vi "Sort queue by Time to next scan.vi"(4 "Queue":T1 {"Scan settings in queue" items=["Regular", "Inverted", "MartinaSettings"]; "Time of the last scan (s)" format="%<%H:%M:%S>t"; "When did you stick it in?" format="%<%H:%M:%S>t"; "Time to next scan (s)" format="%<%H:%M:%S>t"; "Time in rig (s)" format="%<%H:%M:%S>t"}) -> (1 "Queue Out":T1 {"Scan settings in queue" items=["Regular", "Inverted", "MartinaSettings"]; "Time of the last scan (s)" format="%<%H:%M:%S>t"; "When did you stick it in?" format="%<%H:%M:%S>t"; "Time to next scan (s)" format="%<%H:%M:%S>t"; "Time in rig (s)" format="%<%H:%M:%S>t"})   [LabVIEW 2011]
uses:
  Typedefs/Queue.ctl
  Typedefs/Queue cluster.ctl
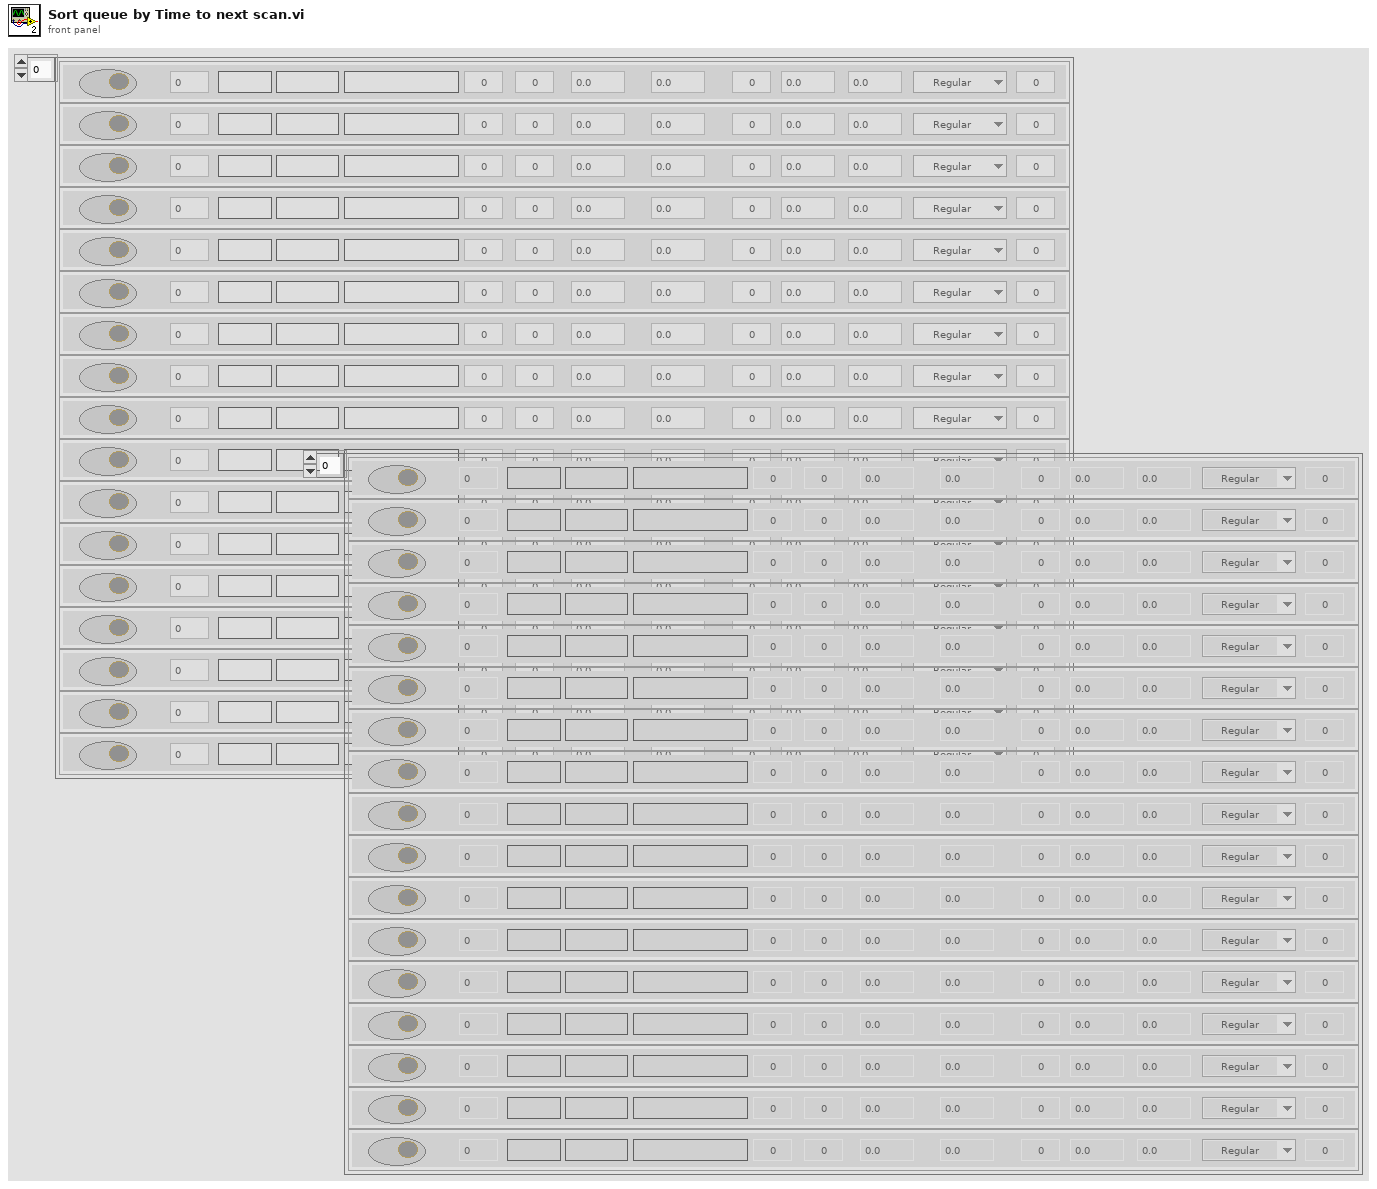
[diagram p1: front panel]
types:
  T1 = typedef "Queue.ctl" = T2[]
  T2 = typedef "Queue cluster.ctl" = cluster{"Measure?":bool, "Area (cm^2)":dbl, "Cell Label":string, "Cell Description":string, "Cell Position":i32, "Time in rig (s)":dbl, "Time to next scan (s)":dbl, "Scan number":dbl, "When did you stick it in?":dbl, "Time between scans (s)":dbl, "Time of the last scan (s)":dbl, "Scan settings in queue":u16, "Sample Holder":dbl, "User Name":string}
  T3 = cluster{"Time to next scan (s)":dbl, "Time of the last scan (s)":dbl, "System Cluster":T2}
  T4 = cluster{"Time to next scan (s)":dbl, "Time of the last scan (s)":dbl, "System Cluster":T2}[]
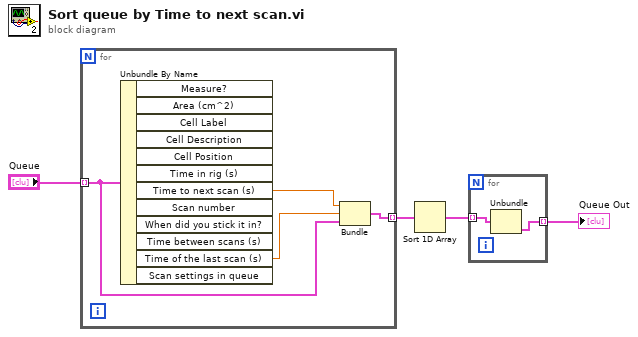
[diagram p0: block diagram]
diagram:
  n1 = for {
    tunnel: "Queue" -> [w8] mode=indexing
    tunnel: [w7] -> w4 mode=indexing
    n2 = Unbundle By Name(w8) -> ("Time to next scan (s)"=w6:dbl, "Time of the last scan (s)"=w5:dbl)  [unwired: 10 out]
    n3 = Bundle("Time to next scan (s)"=w6, "Time of the last scan (s)"=w5, "System Cluster"=w8) -> (w7:T3)  [unwired: 1 in]
  }
  n4 = Sort 1D Array(array=w4) -> (sorted array=w3:T4)
  n5 = for {
    tunnel: w3 -> [w10] mode=indexing
    tunnel: [w9] -> w1 mode=indexing
    n6 = Unbundle(w10) -> ("System Cluster"=w9:T2)  [unwired: 2 out]
  }
  "Queue Out" <- w1
